vi "bmp085_get_calpressure.vi"(8 "error in (no error)":errorcluster, 11 "BMP085 (GY-65) in":refnum<class "BMP085 (GY-65).lvclass">) -> (0 "error out":errorcluster, 2 "p":i32, 3 "BMP085 (GY-65) out":refnum<class "BMP085 (GY-65).lvclass">)   [LabVIEW 2015, in "BMP085 (RT).lvlib" / "BMP085 (GY-65).lvclass"]
uses:
  BMP085 (GY-65).lvclass
  BMP085 (GY-65).lvclass/BMP085 (GY-65).ctl
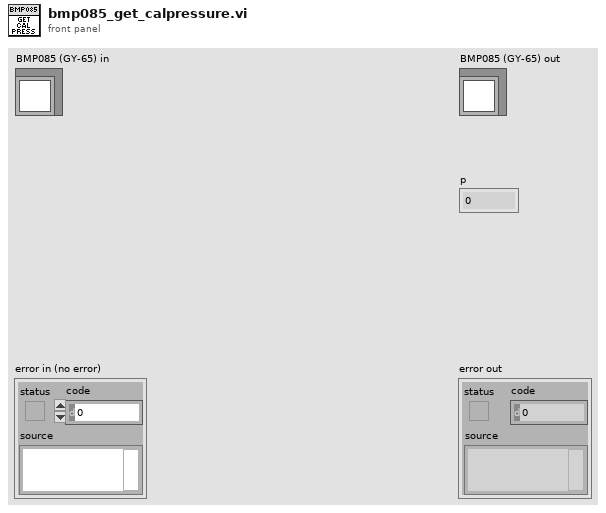
[diagram p1: front panel]
types:
  T1 = enum8{"ultra low power", "standard", "high resolution", "ultra high resolution"}
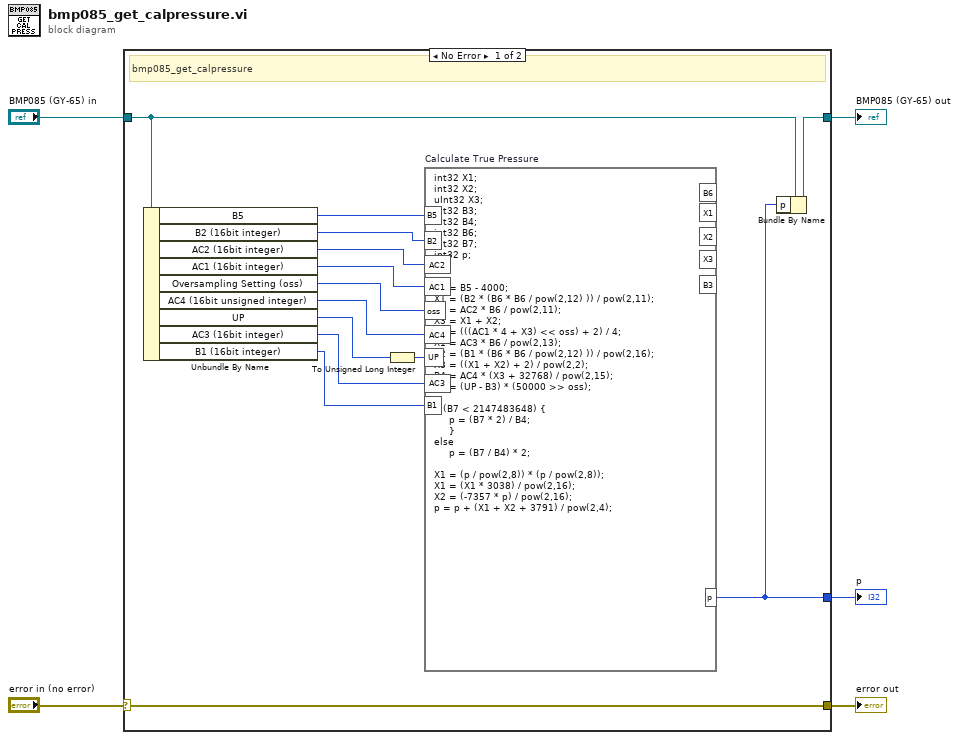
[diagram p0: block diagram]
diagram:
  n1 = case shown="No Error" "error in (no error)" {
    selector: "error in (no error)" -> [w19 w21]
    tunnel: [w19 w21] -> w4
    tunnel: [w7 w20] -> w2
    tunnel: "BMP085 (GY-65) in" -> [w17 w20]
    tunnel: [w6 _] -> w1
    frame No Error {
      # "bmp085_get_calpressure"
      n2 = Unbundle By Name(w17) -> ("B5"=w16:i32, "B2 (16bit integer)"=w15:i16, "AC2 (16bit integer)"=w14:i16, "AC1 (16bit integer)"=w13:i16, "Oversampling Setting (oss)"=w12:T1, "AC4 (16bit unsigned integer)"=w11:u16, "UP"=w10:i32, "AC3 (16bit integer)"=w9:i16, "B1 (16bit integer)"=w8:i16)
      n3 = To Unsigned Long Integer(number=w10) -> (unsigned 32bit integer=w18:u32)
      n4 = formula code="int32 X1;\nint32 X2;\nuInt32 X3;\nint32 B3;\nint32 B4;\nint32 B6;\nint32 B7;\nint32 p;\n\n\nB6 = B5 - 4000;\nX1 = (B2 * (B6 * B6 / pow(2,12) )) / pow(2,11);\nX2 = AC2 * B6 / pow(2,11);\nX3 = X1 + X2;\nB3 = (((AC1 * 4 + X3) << oss) + 2) / 4;\nX1 = AC3 * B6 / pow(2,13);\nX2 = (B1 * (B6 * B6 / pow(2,12) )) / pow(2,16);\nX3 = ((X1 + X2) + 2) / pow(2,2);\nB4 = AC4 * (X3 + 32768) / pow(2,15);\nB7 = (UP - B3) * (50000 >> oss);\n\nif (B7 < 2147483648) {\n     p = (B7 * 2) / B4;\n     }\nelse \n     p = (B7 / B4) * 2;\n\nX1 = (p / pow(2,8)) * (p / pow(2,8));\nX1 = (X1 * 3038) / pow(2,16);\nX2 = (-7357 * p) / pow(2,16);\np = p + (X1 + X2 + 3791) / pow(2,4);" "Calculate True Pressure"("B5"=w16, "AC2"=w14, "B2"=w15, "oss"=w12, "AC1"=w13, "AC4"=w11, "UP"=w18, "AC3"=w9, "B1"=w8) -> ("p"=w6:i32)  [unwired: 5 out]
      n5 = Bundle By Name(cluster=w17, "p"=w6) -> (w7:refnum<class "BMP085 (GY-65).lvclass">)
    }
    frame Error {
    }
  }
  "error out" <- w4
  "BMP085 (GY-65) out" <- w2
  "p" <- w1
